vi "RSZVB Diagram Area Maximize.vi"(8 "error in (no error)":errorcluster {"code" format="%.0x"}, 9 "Diagram Area (1: Maximize)":i32(ring)=1 items=["Restore", "Maximize"], 10 "Window (1)":i32=1, 11 "VISA session":refnum<visa-resource-name>) -> (0 "error out":errorcluster {"code" format="%.0x"}, 3 "dup VISA session":refnum<visa-resource-name>)   [LabVIEW 2011]
doc: "This VI maximizes all diagram areas in the active setup or restores the previous display configuration.\n\nNote(s):\n\nNumber of the diagram area to become the active diagram area. DISPlay:WINDow<Wnd>:MAXimize acts on all diagrams of the current setup, however, the digram no. <Wnd> is displayed on top of the others.\n\nRemote-control command(s):\nDISPlay:WINDow<Wnd>:MAXimize <Boolean>"
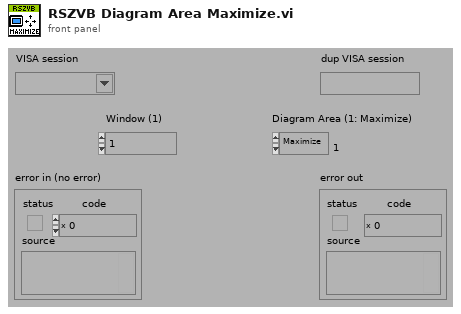
[diagram p1: front panel]
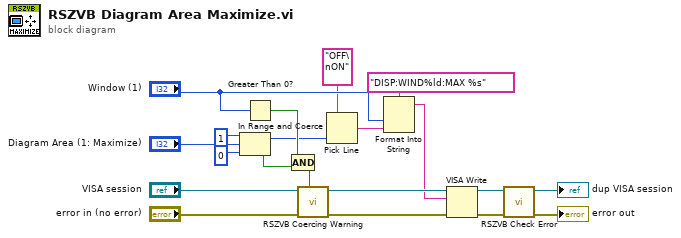
[diagram p0: block diagram]
diagram:
  n1 = In Range and Coerce(upper limit=1, x="Diagram Area (1: Maximize)", lower limit=0) -> (coerced(x)=w2:i32, In Range?=w13:bool)
  n2 = Greater Than 0?(x="Window (1)") -> (x > 0?=w12:bool)
  n3 = Compound Arithmetic op=AND(w12, w13) -> (w11:bool)
  n4 = call "RSZVB Coercing Warning.vi"("In Range?"=w11, "error in (no error)"="error in (no error)", "VISA session"="VISA session") -> ("error out"=w16:errorcluster, "dup VISA session"=w17:refnum<visa-resource-name>)  [unwired: 7 in]
  n5 = Pick Line(multi-line string="OFF\nON", line index=w2) -> (output string=w1:string)  [unwired: 1 in]
  n6 = Format Into String(format string="DISP:WIND%ld:MAX %s", "Window (1)", w1) -> (resulting string=w10:string)  [unwired: 2 in, 1 out]
  n7 = VISA Write(VISA resource name=w17, write buffer=w10, error in (no error)=w16) -> (VISA resource name out=w14:refnum<visa-resource-name>, error out=w15:errorcluster)  [unwired: 1 out]
  n8 = call "RSZVB Check Error.vi"("error in (no error)"=w15, "VISA session"=w14) -> ("error out"=→"error out":errorcluster, "dup VISA session"=→"dup VISA session":refnum<visa-resource-name>)  [unwired: 8 in]
